vi "Average_Precision_Score.vi"(8 "error in (no error)":errorcluster caption="entrée d'erreur (pas d'erreur)", 9 "y_score":string[][](array[string]), 10 "y_true":string[][](array[string]), 11 "average_precision_score":T1={"average"="macro", "pos_label"={"dtype_pos_label"="int", "pos_label"="1"}, "sample_weight"=[]}) -> (0 "error out":errorcluster caption="sortie d'erreur", 3 "String Data":string)   [LabVIEW 2020]
doc: "Compute average precision (AP) from prediction scores\n\nAP summarizes a precision-recall curve as the weighted mean of precisions achieved at each threshold, with the increase in recall from the previous threshold used as the weight :\n\n AP = SUM(R_n - R_(n-1))P_n \n\nwhere Pn and Rn are the precision and recall at the nth threshold [1]. This implementation is not interpolated and is different from computing the area under the precision-recall curve with the trapezoidal rule, which uses linear interpolation and can be too optimistic.\n\nNote: this implementation is restricted to the binary classification task or multilabel classification task.\n\n\nParameters : \n\n- y_true : array, shape = [n_samples] or [n_samples, n_classes]\nTrue binary labels or binary label indicators.\n\n- y_score : array, shape = [n_samples] or [n_samples, n_classes]\nTarget scores, can either be probability estimates of the positive class, confidence values, or non-thresholded measure of decisions (as returned by “decision_function” on some classifiers).\n\n- average : string, [None, ‘micro’, ‘macro’ (default), ‘samples’, ‘weighted’]\nIf None, the scores for each class are returned. Otherwise, this determines the type of averaging performed on the data:\n\n'micro':\nCalculate metrics globally by considering each element of the label indicator matrix as a label.\n\n'macro':\nCalculate metrics for each label, and find their unweighted mean. This does not take label imbalance into account.\n\n'weighted':\nCalculate metrics for each label, and find their average, weighted by support (the number of true instances for each label).\n\n'samples':\nCalculate metrics for each instance, and find their average.\n\nWill be ignored when y_true is binary.\n\n- pos_label : int or str (default=1)\nThe label of the positive class. Only applied to binary y_true. For multilabel-indicator y_true, pos_label is fixed to 1.\n\n- sample_weight : array-like of shape (n_samples,), default=None\nSample weights.\n\nReturns : \n\n-average_precision : float"
uses:
  Average_Precision_Score.lvclass
panel:
  out "Average_Precision_Score.lvclass":refnum<class "Average_Precision_Score.lvclass">
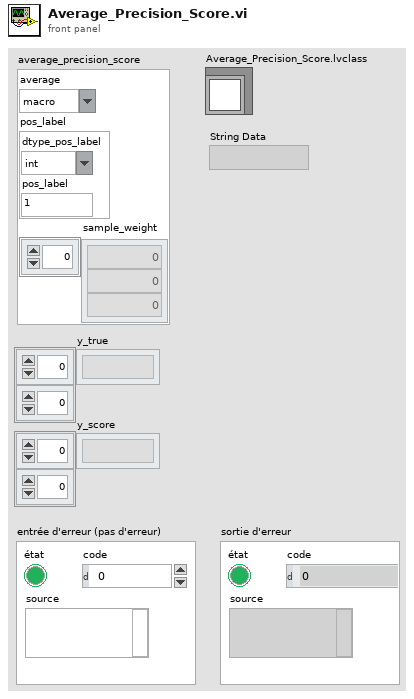
[diagram p1: front panel]
types:
  T1 = cluster{"average":string, "pos_label":cluster{"dtype_pos_label":string, "pos_label":string}, "sample_weight":dbl[]}
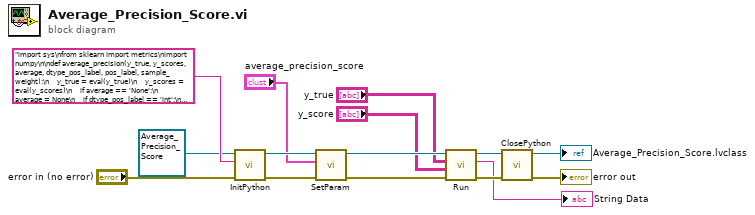
[diagram p0: block diagram]
diagram:
  n1 = call-dynamic "InitPython.vi"("error in (no error)"="error in (no error)", "Python Instruction"="import sys\nfrom sklearn import metrics\nimport numpy\n\ndef average_precision(y_true, y_scores, average, dtype_pos_label, pos_label, sample_weight):\n    y_true = eval(y_true)\n    y_scores = eval(y_scores)\n    if average == 'None':\n        average = None\n    if dtype_pos_label == 'int':\n        pos_label = eval(pos_label)\n    if sample_weight == []:\n        sample_weight = None\n    try:\n        average_precision_score = metrics.average_precision_score(y_true, y_scores, average, pos_label, sample_weight)\n        average_precision_score = average_precision_score.tolist()\n        return str(average_precision_score)\n    except:\n        erreur = sys.exc_info()\n        typerr = u\"%s\" % (erreur[0])\n        typerr = typerr[typerr.find(\"'\")+1:typerr.rfind(\"'\")]\n        msgerr = u\"%s\" % (erreur[1])\n        message = str('/!\\\\ {0} : {1}'. format(typerr,msgerr))\n        return message", "Scikit-learn en entrée"=refnum<class "Average_Precision_Score.lvclass"> refnum ("Average_Precision_Score.lvclass")) -> ("error out"=w10:errorcluster, "Scikit-learn en sortie"=w11:refnum<class "Average_Precision_Score.lvclass">)  [unwired: 7 in]
  n2 = call-dynamic "SetParam.vi"("error in (no error)"=w10, "average_precision_score"="average_precision_score", "Average_Precision_Score.lvclass"=w11) -> ("error out"=w4:errorcluster, "Average_Precision_Score.lvclass"=w8:refnum<class "Average_Precision_Score.lvclass">)  [unwired: 7 in]
  n3 = call-dynamic "Run.vi"("error in (no error)"=w4, "y_score"="y_score", "y_true"="y_true", "Average_Precision_Score.lvclass"=w8) -> ("error out"=w6:errorcluster, "String Data"=→"String Data":string, "Average_Precision_Score.lvclass"=w7:refnum<class "Average_Precision_Score.lvclass">)  [unwired: 5 in]
  n4 = call-dynamic "ClosePython.vi"("error in (no error)"=w6, "Scikit-learn en entrée"=w7) -> ("error out"=→"error out":errorcluster, "Scikit-learn en sortie"=→"Average_Precision_Score.lvclass":refnum<class "Average_Precision_Score.lvclass">)  [unwired: 8 in]
